vi "Sel Chassis 0.vi"(8 "error in (no error)":errorcluster, 11 "Cfg Grandmaster in":refnum<class "Cfg Grandmaster.lvclass">) -> (0 "error out":errorcluster, 3 "Cfg Grandmaster out":refnum<class "Cfg Grandmaster.lvclass">)   [LabVIEW 2018, in "Configuration Grandmaster.lvlib" / "Cfg Grandmaster.lvclass"]
uses:
  Cfg Grandmaster.lvclass
  Cfg Grandmaster.lvclass/Cfg Grandmaster.ctl
  Class Chassis BOM/Chassis BOM.lvclass/Chassis BOM.ctl
  Class Chassis BOM/Read Chassis Alias.vi
  Class Chassis BOM/Chassis BOM.lvclass
  Class FP Ctrls/FP Controls.lvclass
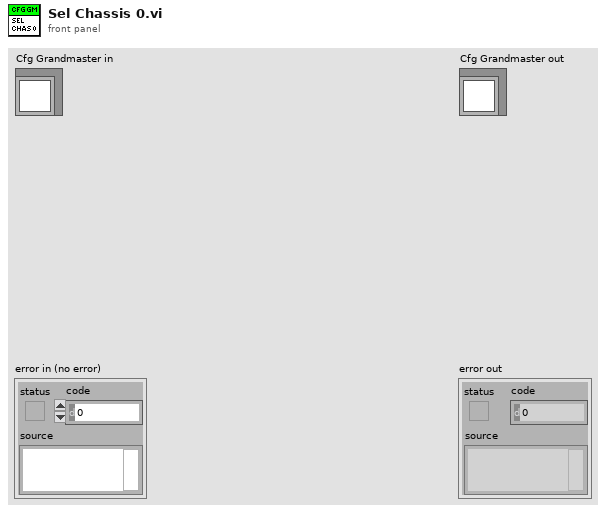
[diagram p1: front panel]
types:
  T1 = typedef "ge_Cfg wChassis.ctl" = cluster{"Chassis BOM":refnum<class "Chassis BOM.lvclass">, "Chassis Cfg":refnum<class "ChassisCfg.lvclass">, "Chassis Tasks":refnum<class "Chassis Tasks.lvclass">, "HW Error":bool, "Unsvd Chgs?":bool}
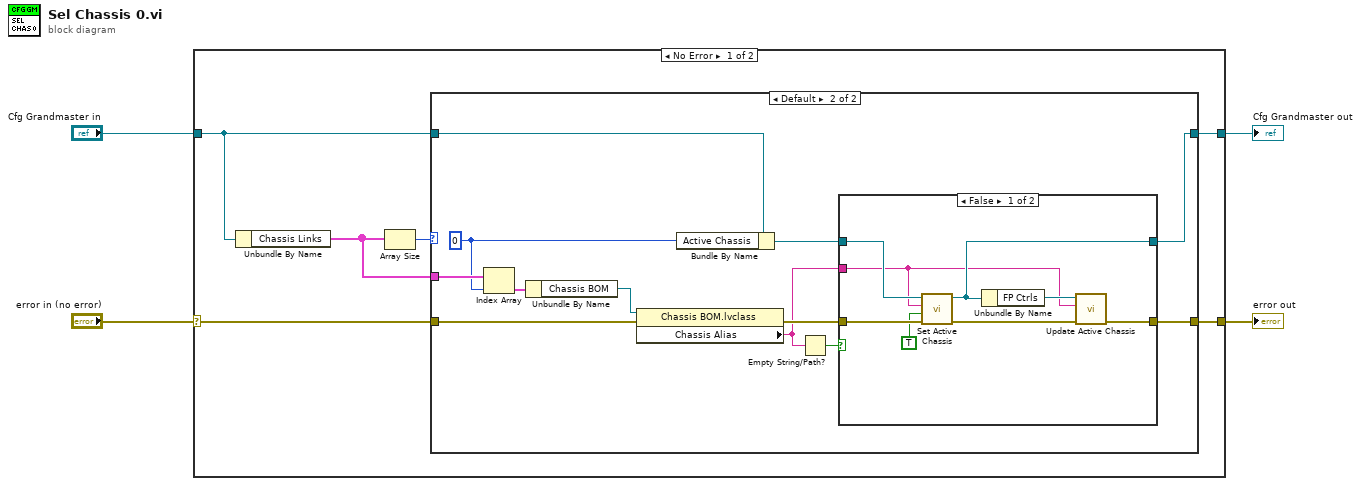
[diagram p0: block diagram]
diagram:
  n1 = case shown="No Error" "error in (no error)" {
    selector: "error in (no error)" -> [w8 w36]
    tunnel: [w7 w36] -> w3
    tunnel: [w5 w35] -> w1
    tunnel: "Cfg Grandmaster in" -> [w6 w35]
    frame No Error {
      n2 = Unbundle By Name(w6) -> ("Chassis Links"=w9:T1[])
      n3 = Array Size(array=w9) -> (size(s)=w10:i32)
      n4 = case shown="Default" w10 {
        tunnel: w9 -> [_ w24]
        tunnel: w8 -> [w12 w20]
        tunnel: [w12 w22] -> w7
        tunnel: w6 -> [w11 w16]
        tunnel: [w11 w13] -> w5
        frame 0 {
        }
        frame Default {
          w15 = 0
          n5 = Index Array(array=w24, index=w15) -> (element=w17:T1)
          n6 = Unbundle By Name(w17) -> ("Chassis BOM"=w21:refnum<class "Chassis BOM.lvclass">)
          n7 = property class="Chassis BOM.lvclass"(reference=w21, error in=w20) -> (error out=w19:errorcluster, "Chassis Alias"=w18:string)  [unwired: 1 out]
          n8 = Bundle By Name(cluster=w16, "Active Chassis"=w15) -> (w14:refnum<class "Cfg Grandmaster.lvclass">)
          n9 = Empty String/Path?(string/path=w18) -> (empty?=w23:bool)
          n10 = case shown="False" w23 {
            tunnel: w18 -> [w25 _]
            tunnel: w19 -> [w32 w34]
            tunnel: [w28 w34] -> w22
            tunnel: w14 -> [w30 w33]
            tunnel: [w27 w33] -> w13
            frame False {
              n11 = call "Set Active Chassis.vi"("error in (no error)"=w32, "Rfrsh GUI? (T)"=TRUE ("Rfrsh GUI?"), "Chassis Name"=w25, "Cfg Grandmaster in"=w30) -> ("error out"=w29:errorcluster, "Cfg Grandmaster out"=w27:refnum<class "Cfg Grandmaster.lvclass">)  [unwired: 6 in]
              n12 = Unbundle By Name(w27) -> ("FP Ctrls"=w26:refnum<class "FP Controls.lvclass">)
              n13 = call "Update Active Chassis.vi"("error in (no error)"=w29, "Active Chassis"=w25, "FP Controls in"=w26) -> ("error out"=w28:errorcluster)  [unwired: 7 in, 1 out]
            }
            frame True {
            }
          }
        }
      }
    }
    frame Error {
    }
  }
  "error out" <- w3
  "Cfg Grandmaster out" <- w1
